vi "_scriptEditor.Input Candidates.vi"(11 "Selection":T1) -> (3 "Array":string[](array[string]))   [LabVIEW 2017]
uses:
  CSM Part Property.ctl
  Single-Line Selection Type.ctl
  _csmHelper/API with lvcsm Support/CSM-Helper API with lvcsm Support.lvlib
  Communicable State Machine.lvlib
  _Shared/CSM Shared.lvlib
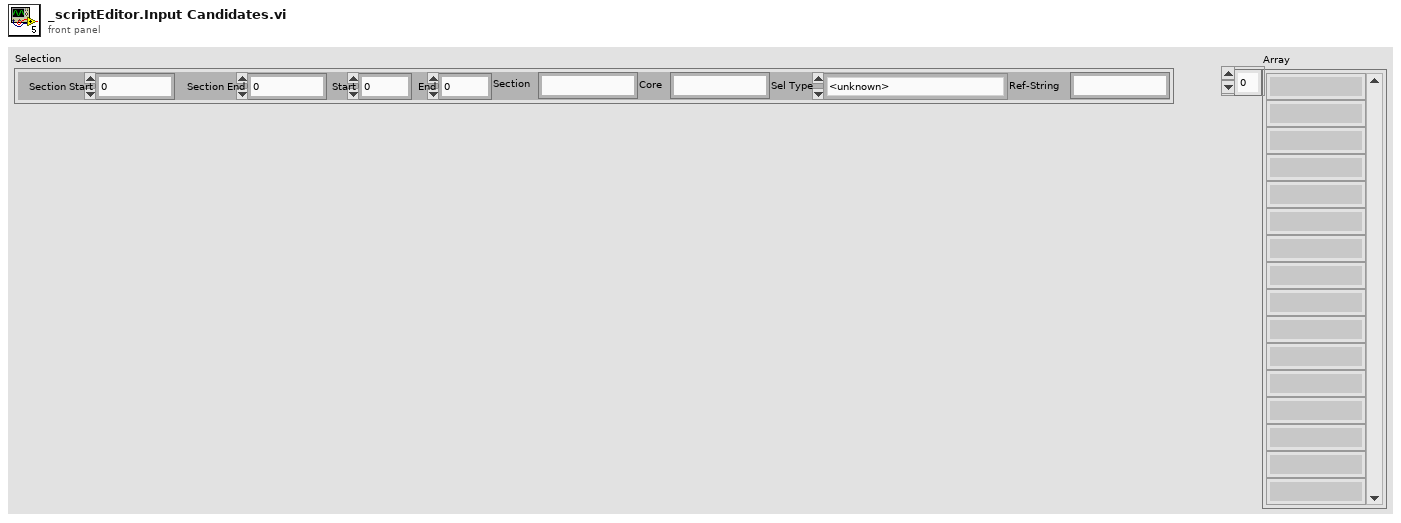
[diagram p1: front panel]
types:
  T1 = typedef "CSM Part Property.ctl" = cluster{"Section Start":u32, "Section End":u32, "Start":u32, "End":u32, "Section":string, "Core":string, "Sel Type":T2, "Ref-String":string}
  T2 = typedef "Single-Line Selection Type.ctl" = enum16{"<unknown>", "Reg-SourceSignal", "Reg-@Seperator", "Reg-ArgSymbol", "Reg-TargetAPI", "Reg-Module", "Reg-Symbol", "Reg-Oper", "Msg-State", "Msg-Arg", "Msg-ArgSymbol", "Msg-Symbol", "Msg-Module", "Broadcast-Signal", "Broadcast-ArgSymbol", "Broadcast-Arg", "Broadcast-Symbol", "Broadcast-Oper", "Comment-Symbol", "Comment-Content"}
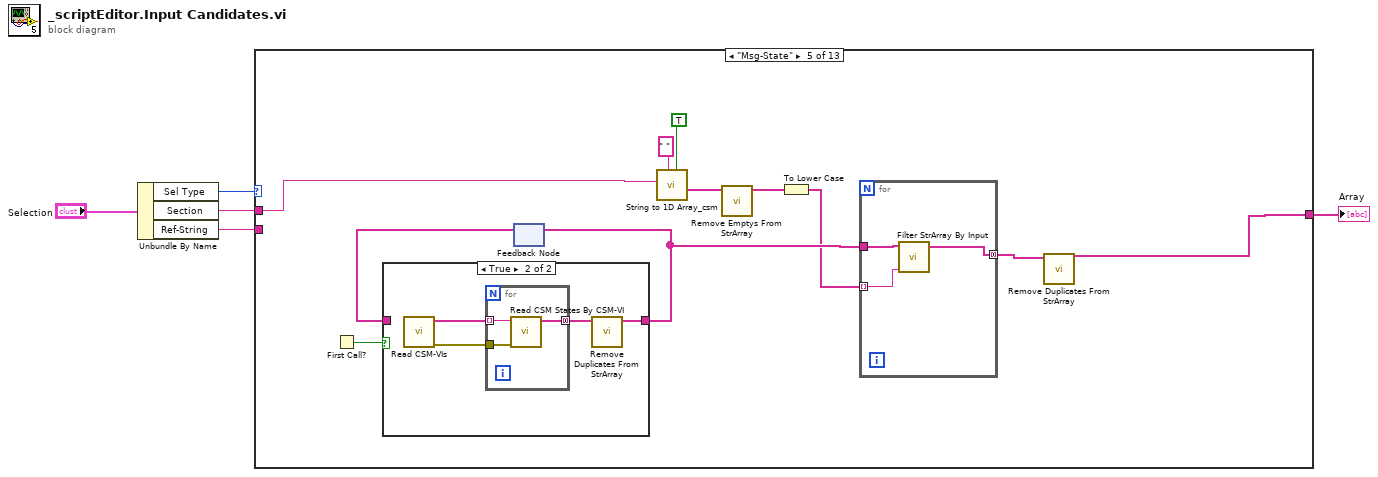
[diagram p0: block diagram]
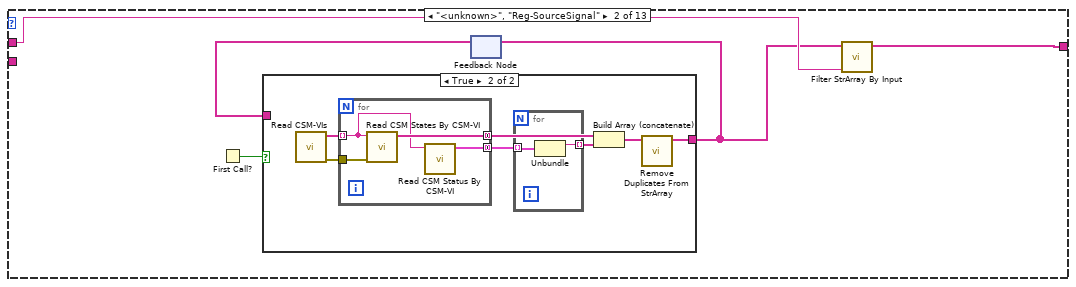
[diagram p3: hidden frame]
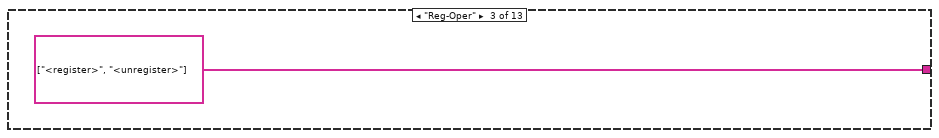
[diagram p5: hidden frame]
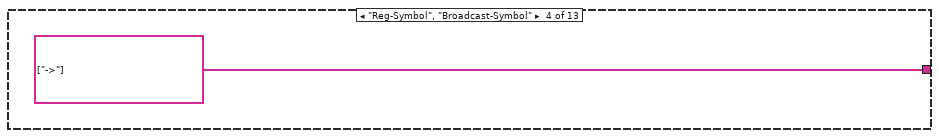
[diagram p6: hidden frame]
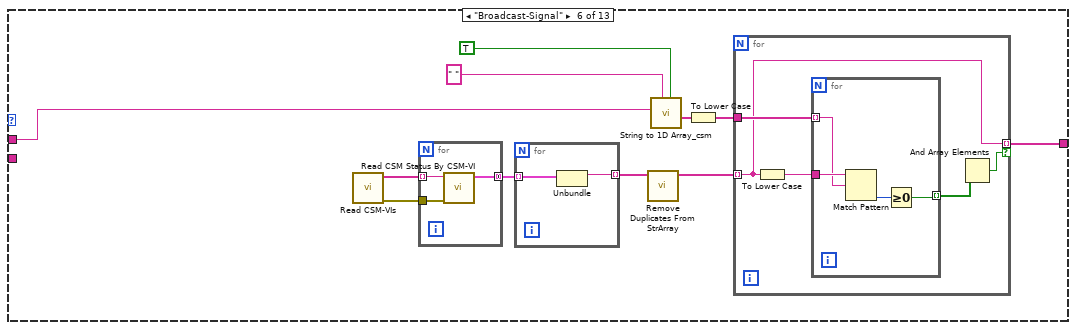
[diagram p8: hidden frame]
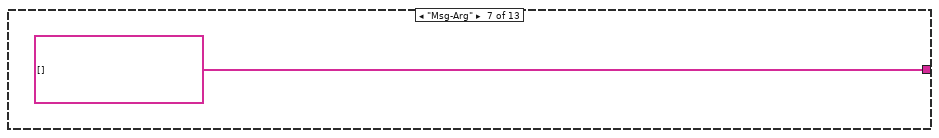
[diagram p9: hidden frame]
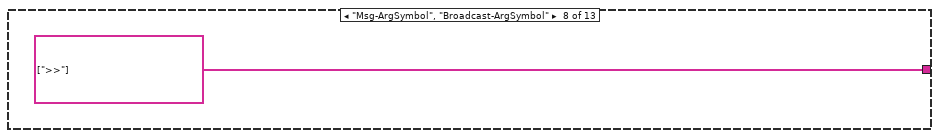
[diagram p10: hidden frame]
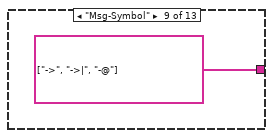
[diagram p11: hidden frame]
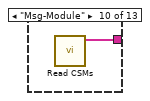
[diagram p12: hidden frame]
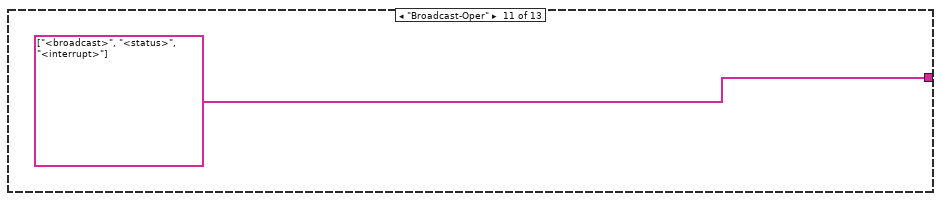
[diagram p13: hidden frame]
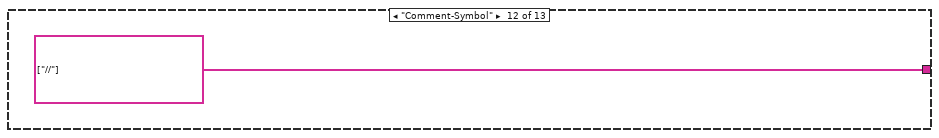
[diagram p14: hidden frame]
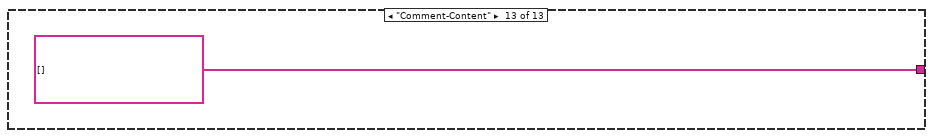
[diagram p15: hidden frame]
diagram:
  n1 = Unbundle By Name("Selection") -> ("Sel Type"=w2:T2, "Section"=w5:string, "Ref-String"=w4:string)
  n2 = case shown="\"Msg-State\"" w2 {
    tunnel: [_ w10 string[] ["<register>", "<unregister>"] string[] ["->"] w33 w54 string[] [] string[] [">>"] string[] ["->", "->|", "-@"] w77 string[] ["<broadcast>", "<status>", "<interrupt>"] string[] ["//"] string[] []] -> w3
    tunnel: w4 -> [_ _ _ _ _ _ _ _ _ _ _ _ _]
    tunnel: w5 -> [_ w9 _ _ w29 w57 _ _ _ _ _ _ _]
    frame Default {
    }
    frame "<unknown>", "Reg-SourceSignal" {
      n3 = First Call?() -> (First Call?: T/F=w7:bool)
      n4 = feedback #1() -> (w6:string[])  [unwired: 1 in]
      n5 = case shown="True" w7 {
        tunnel: [w11 w12] -> w8
        tunnel: w6 -> [w11 _]
        frame False {
        }
        frame True {
          n6 = call "Read CSM-VIs.vi"() -> ("Error Out"=w17:errorcluster, "Array"=w16:string[])  [unwired: 10 in]
          n7 = for {
            tunnel: [w24] -> w18 mode=concatenating
            tunnel: w17 -> [w23]
            tunnel: w16 -> [w22] mode=indexing
            tunnel: [w21] -> w14 mode=concatenating
            n8 = call "Read CSM States By CSM-VI.vi"("Error In"=w23, "CSM VI"=w22) -> ("Array"=w24:string[])  [unwired: 8 in, 1 out]
            n9 = call "Read CSM Status By CSM-VI.vi"("CSM VI"=w22) -> ("Array 3"=w21:cluster{"Status":string, "InState":string}[])  [unwired: 9 in, 1 out]
          }
          n10 = for {
            tunnel: w14 -> [w20] mode=indexing
            tunnel: [w19] -> w13 mode=indexing
            n11 = Unbundle(w20) -> ("Status"=w19:string)  [unwired: 1 out]
          }
          n12 = Build Array (concatenate)(w18, w13) -> (w15:string[])
          n13 = call "Remove Duplicates From StrArray.vi"("StrArray In"=w15) -> ("StrArray"=w12:string[])  [unwired: 9 in, 1 out]
        }
      }
      n14 = feedback-in #1(w8) -> ()
      n15 = call "Filter StrArray By Input.vi"("Filter String"=w9, "Array In"=w8) -> ("Array"=w10:string[])  [unwired: 9 in]
    }
    frame "Reg-Oper" {
    }
    frame "Reg-Symbol", "Broadcast-Symbol" {
    }
    frame "Msg-State" {
      n16 = First Call?() -> (First Call?: T/F=w37:bool)
      n17 = feedback #2() -> (w36:string[])  [unwired: 1 in]
      n18 = case shown="True" w37 {
        tunnel: [w41 w42] -> w35
        tunnel: w36 -> [w41 _]
        frame False {
        }
        frame True {
          n19 = call "Read CSM-VIs.vi"() -> ("Error Out"=w45:errorcluster, "Array"=w44:string[])  [unwired: 10 in]
          n20 = for {
            tunnel: [w48] -> w43 mode=concatenating
            tunnel: w45 -> [w47]
            tunnel: w44 -> [w46] mode=indexing
            n21 = call "Read CSM States By CSM-VI.vi"("Error In"=w47, "CSM VI"=w46) -> ("Array"=w48:string[])  [unwired: 8 in, 1 out]
          }
          n22 = call "Remove Duplicates From StrArray.vi"("StrArray In"=w43) -> ("StrArray"=w42:string[])  [unwired: 9 in, 1 out]
        }
      }
      n23 = feedback-in #2(w35) -> ()
      n24 = call "String to 1D Array_csm.vi"("ignore duplicate delimiters? (F=No)"=TRUE, "delimiter (Tab)"=" ", "string"=w29) -> ("Array of Strings"=w30:string[])  [unwired: 8 in]
      n25 = call "Remove Emptys From StrArray.vi"("Array In"=w30) -> ("Array Out"=w27:string[])  [unwired: 10 in]
      n26 = To Lower Case(string=w27) -> (all lower case string=w28:string[])
      n27 = for {
        tunnel: w35 -> [w40]
        tunnel: [w38] -> w34 mode=concatenating
        tunnel: w28 -> [w39] mode=indexing
        n28 = call "Filter StrArray By Input.vi"("Filter String"=w39, "Array In"=w40) -> ("Array"=w38:string[])  [unwired: 9 in]
      }
      n29 = call "Remove Duplicates From StrArray.vi"("StrArray In"=w34) -> ("StrArray"=w33:string[])  [unwired: 9 in, 1 out]
    }
    frame "Broadcast-Signal" {
      n30 = call "Read CSM-VIs.vi"() -> ("Error Out"=w59:errorcluster, "Array"=w58:string[])  [unwired: 10 in]
      n31 = for {
        tunnel: [w73] -> w51 mode=concatenating
        tunnel: w59 -> [w72]
        tunnel: w58 -> [w71] mode=indexing
        n32 = call "Read CSM Status By CSM-VI.vi"("Error In"=w72, "CSM VI"=w71) -> ("Array 3"=w73:cluster{"Status":string, "InState":string}[])  [unwired: 8 in, 1 out]
      }
      n33 = for {
        tunnel: w51 -> [w61] mode=indexing
        tunnel: [w60] -> w50 mode=indexing
        n34 = Unbundle(w61) -> ("Status"=w60:string)  [unwired: 1 out]
      }
      n35 = call "Remove Duplicates From StrArray.vi"("StrArray In"=w50) -> ("StrArray"=w49:string[])  [unwired: 9 in, 1 out]
      n36 = call "String to 1D Array_csm.vi"("ignore duplicate delimiters? (F=No)"=TRUE, "delimiter (Tab)"=" ", "string"=w57) -> ("Array of Strings"=w56:string[])  [unwired: 8 in]
      n37 = To Lower Case(string=w56) -> (all lower case string=w55:string[])
      n38 = for {
        tunnel: w49 -> [w64] mode=indexing
        tunnel: w55 -> [w65]
        tunnel: [w64] -> w54 mode=indexing if=w63
        n39 = To Lower Case(string=w64) -> (all lower case string=w66:string)
        n40 = for {
          tunnel: w66 -> [w70]
          tunnel: [w68] -> w62 mode=indexing
          tunnel: w65 -> [w67] mode=indexing
          n41 = Match Pattern(string=w70, regular expression=w67) -> (offset past match=w69:i32)  [unwired: 1 in, 3 out]
          n42 = Greater Or Equal To 0?(x=w69) -> (x >= 0?=w68:bool)
        }
        n43 = And Array Elements(Boolean array=w62) -> (logical AND=w63:bool)
      }
    }
    frame "Msg-Arg" {
    }
    frame "Msg-ArgSymbol", "Broadcast-ArgSymbol" {
    }
    frame "Msg-Symbol" {
    }
    frame "Msg-Module" {
      n44 = call "Read CSMs.vi"() -> ("Array"=w77:string[])  [unwired: 10 in, 1 out]
    }
    frame "Broadcast-Oper" {
    }
    frame "Comment-Symbol" {
    }
    frame "Comment-Content" {
    }
  }
  "Array" <- w3
